vi "Protokoll anzeigen.vi"(11 "String":string) -> ()   [LabVIEW 2010]
panel:
  out "error out":errorcluster caption="Fehler (Ausgang)"
  out "String 2":string
  in  "speichern":bool
  in  "ok":bool
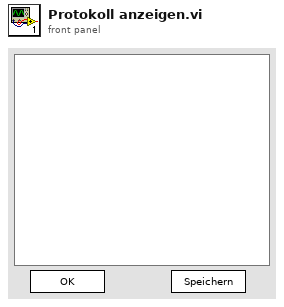
[diagram p1: front panel]
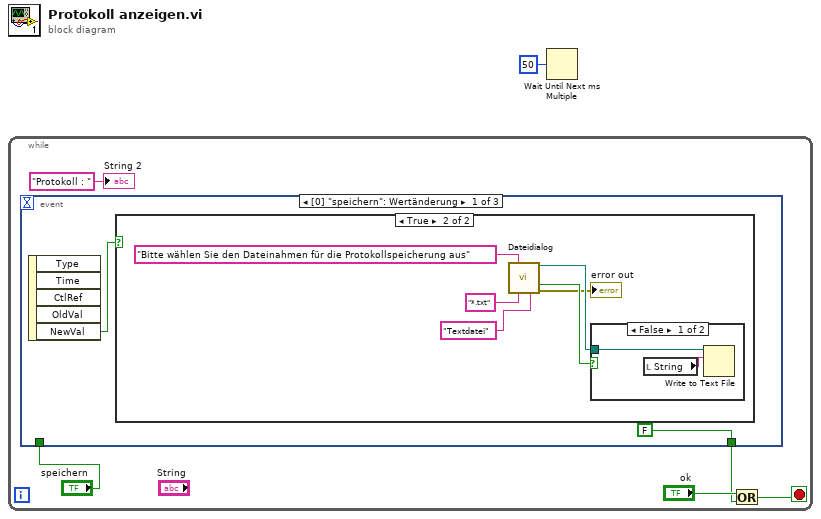
[diagram p0: block diagram]
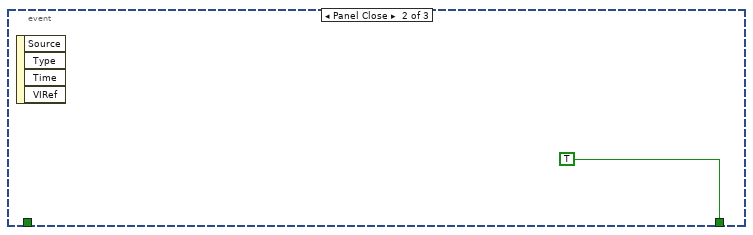
[diagram p4: hidden frame]
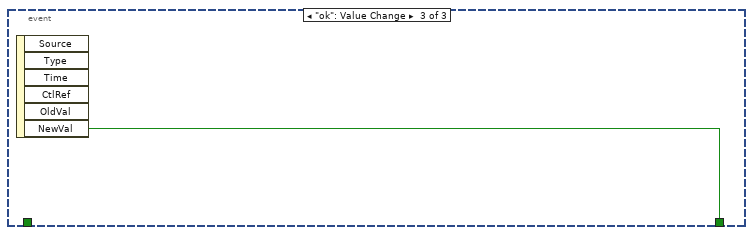
[diagram p5: hidden frame]
diagram:
  n1 = while {
    stop <- w3 stop-if-true
    n2 = event shown="[0] \"speichern\": Wertänderung" {
      selector: _ -> [_ _ _]
      dyn-events: _ -> [_ _ _]
      timeout: _ -> [_ _ _]
      tunnel: "speichern" -> [_ _ _]
      tunnel: [FALSE TRUE w18] -> w2
      event "speichern": Value Change {
        n3 = event-data() -> ("NewVal"=w8:bool)  [unwired: 5 out]
        n4 = case shown="TRUE" w8 {
          frame False {
          }
          frame True {
            n5 = call "Dateidialog"("prompt"="Bitte wählen Sie den Dateinahmen für die Protokollspeicherung aus", "pattern (all files)"="*.txt", "pattern label"="Textdatei") -> ("selected path"=w10:path, "cancelled"=w11:bool, "error out"=→"error out":errorcluster)  [unwired: 4 in, 6 out]
            n6 = case shown="FALSE" w11 {
              tunnel: w10 -> [w15 _]
              frame False {
                n7 = local read "String"() -> (w16:string)
                n8 = Write to Text File(file (use dialog)=w15, text=w16) -> ()  [unwired: 1 in, 4 out]
              }
              frame True {
              }
            }
          }
        }
      }
      event Panel Close {
        n9 = event-data() -> ()  [unwired: 5 out]
      }
      event "ok": Value Change {
        n10 = event-data() -> ("NewVal"=w18:bool)  [unwired: 6 out]
      }
    }
    n11 = Or(x="ok", y=w2) -> (x .or. y?=w3:bool)
    "String 2" <- "Protokoll : " ("String 2")
  }
  n12 = Wait Until Next ms Multiple(millisecond multiple=u32 50 ("Vielfache von ms")) -> ()  [unwired: 1 out]
